vi "Module Loop.vi"(8 "error in (no error)":errorcluster, 11 "GenericGuiAI in":refnum<class "GenericGuiAI.lvclass">) -> (0 "error out":errorcluster, 3 "GenericGuiAI out":refnum<class "GenericGuiAI.lvclass">)   [LabVIEW 2020, in "VolatusDAQGenericGUI.lvlib" / "GenericGuiAI.lvclass"]
uses:
  GenericGuiAI.lvclass
  C:/dev/lv20CE/relink/lv-volatus/Volatus/Module/Module.lvclass
  Volatus/Module/Module.lvclass/Module.ctl
  Volatus/MessageQ/MessageQ.lvclass/MessageQ.ctl
  Volatus/Module/Module.lvclass
  <vilib>/Utility/error.llb/Error Cluster From Error Code.vi
  Volatus/MessageQ/MessageQ.lvclass
panel:
  in  "Tree":string(tree)
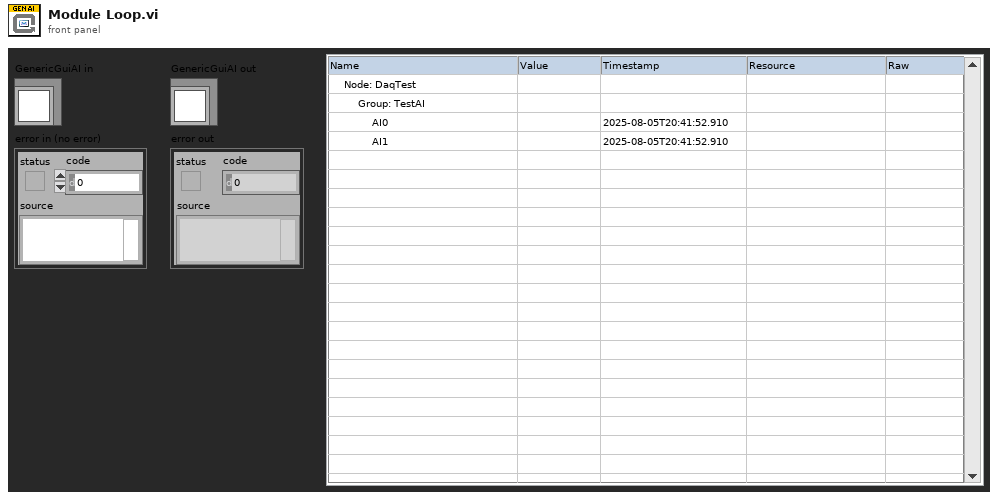
[diagram p1: front panel]
types:
  T1 = enum32{"Invalid", "Standard", "Closed", "Hidden", "Minimized", "Maximized"}
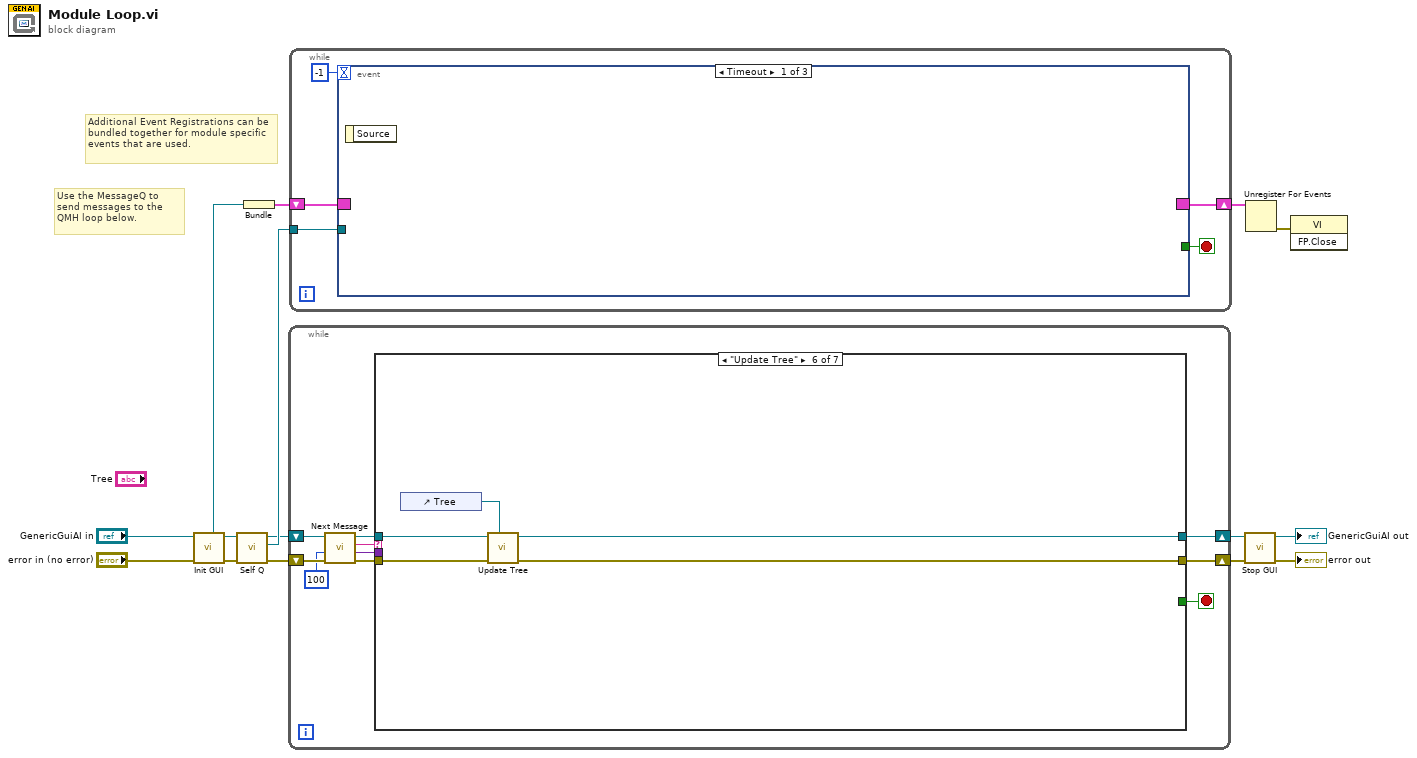
[diagram p0: block diagram]
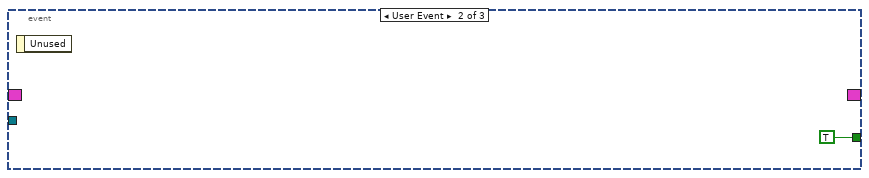
[diagram p2: hidden frame]
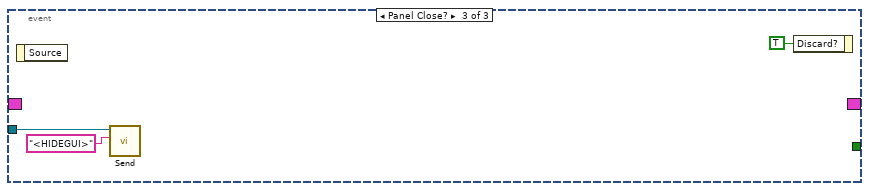
[diagram p3: hidden frame]
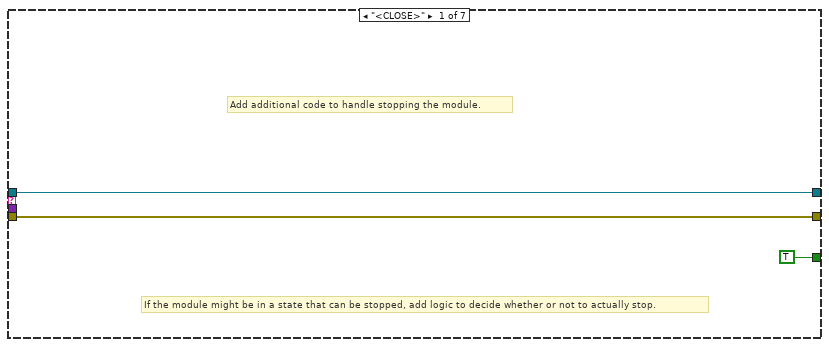
[diagram p4: hidden frame]
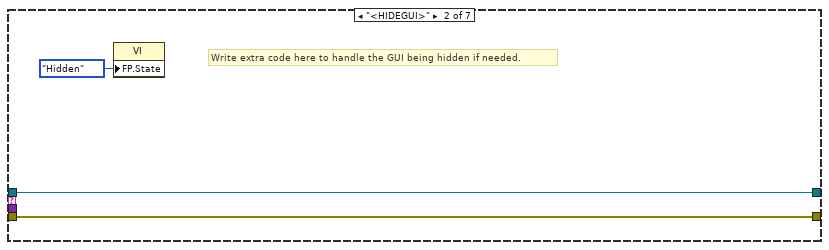
[diagram p5: hidden frame]
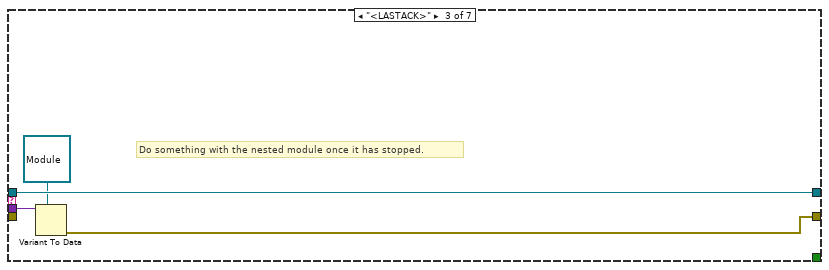
[diagram p6: hidden frame]
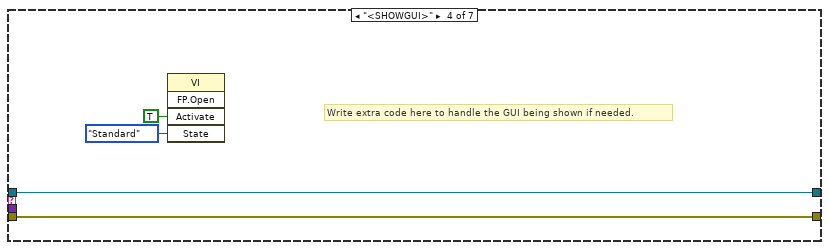
[diagram p7: hidden frame]
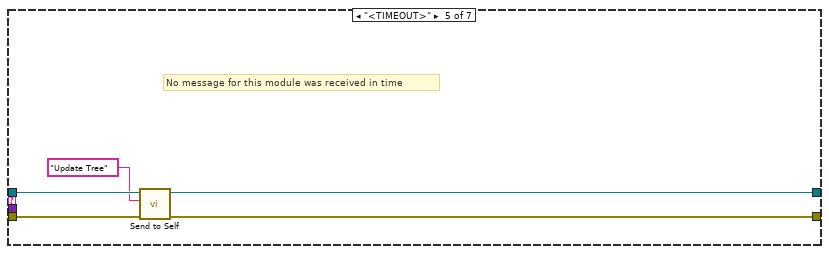
[diagram p8: hidden frame]
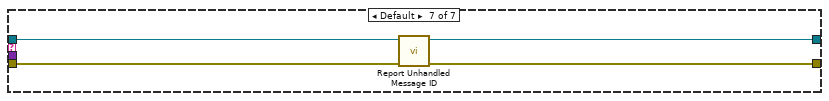
[diagram p9: hidden frame]
diagram:
  # "Additional Event Registrations can be bundled together for module specific events that are used."
  # "Use the MessageQ to send messages to the QMH loop below."
  n1 = call "Init GUI.vi"("Module in"="GenericGuiAI in") -> ("Module out"=w7:refnum<class "GenericGuiAI.lvclass">, "Event Reg"=w12:refnum<event-registration>)  [unwired: 9 in]
  n2 = call "Self Q.vi"("Module in"=w7) -> ("Self Q"=w6:refnum<class "MessageQ.lvclass">, "Module out"=w5:refnum<class "GenericGuiAI.lvclass">)  [unwired: 9 in]
  n3 = Bundle("Event Reg"=w12) -> (w8:cluster{"Event Reg":refnum<event-registration>})  [unwired: 1 in]
  n4 = while {
    shift-right: [w18] -> w10
    shift-left: w5 -> [w23]
    shift-right: [w17] -> w11
    shift-left: "error in (no error)" -> [w22]
    stop <- w16 stop-if-true
    n5 = call "Next Message.vi"("error in (no error)"=w22, "Timeout ms (-1)"=100, "Module in"=w23) -> ("error out"=w21:errorcluster, "Data"=w15:variant, "ID"=w20:string, "Module out"=w19:refnum<class "GenericGuiAI.lvclass">)  [unwired: 5 in]
    n6 = case shown="\"Update Tree\"" w20 {
      tunnel: w21 -> [w24 w28 _ w36 w42 w47 w51]
      tunnel: w19 -> [w25 w29 w33 w37 w40 w45 w49]
      tunnel: [w25 w29 w33 w37 w39 w44 w48] -> w18
      tunnel: [w24 w28 w30 w36 w41 w46 w50] -> w17
      tunnel: [TRUE _ _ _ _ _ _] -> w16
      tunnel: w15 -> [_ _ w32 _ _ _ _]
      frame "<CLOSE>" {
        # "If the module might be in a state that can be stopped, add logic to decide whether or not to actually stop."
        # "Add additional code to handle stopping the module."
      }
      frame "<HIDEGUI>" {
        # "Write extra code here to handle the GUI being hidden if needed."
        n7 = property class="VI"("FP.State"=T1."Hidden" ("Front Panel Window:State")) -> ()  [unwired: 2 in, 2 out]
      }
      frame "<LASTACK>" {
        # "Do something with the nested module once it has stopped."
        n8 = Variant To Data(type=refnum<class "Module.lvclass"> refnum ("Volatus:Module"), Variant=w32) -> (error out=w30:errorcluster)  [unwired: 1 in, 1 out]
      }
      frame "<SHOWGUI>" {
        # "Write extra code here to handle the GUI being shown if needed."
        n9 = invoke class="VI" method="FP.Open"("Activate"=TRUE ("Activate?"), "State"=T1."Standard") -> ()  [unwired: 3 in, 5 out]
      }
      frame "<TIMEOUT>" {
        # "No message for this module was received in time"
        n10 = call "Send to Self.vi"("error in (no error)"=w42, "Message ID"="Update Tree", "Module in"=w40) -> ("error out"=w41:errorcluster, "Module out"=w39:refnum<class "GenericGuiAI.lvclass">)  [unwired: 7 in]
      }
      frame "Update Tree" {
        n11 = control-ref of="Tree"() -> (w43:refnum<vi>)
        n12 = call "Update Tree.vi"("Tree"=w43, "error in (no error)"=w47, "GenericGuiAI in"=w45) -> ("error out"=w46:errorcluster, "GenericGuiAI out"=w44:refnum<class "GenericGuiAI.lvclass">)  [unwired: 7 in]
      }
      frame Default {
        n13 = call "Report Unhandled Message ID.vi"("error in (no error)"=w51, "Module in"=w49) -> ("error out"=w50:errorcluster, "Module out"=w48:refnum<class "GenericGuiAI.lvclass">)  [unwired: 8 in]
      }
    }
  }
  n14 = while {
    tunnel: w6 -> [w56]
    shift-right: [w54] -> w9
    shift-left: w8 -> [w55]
    stop <- w53 stop-if-true
    n15 = event shown="[0] Timeout" {
      selector: w55 -> [_ _ _]
      dyn-events: [_ _ _] -> w54
      timeout: -1 -> [_ _ _]
      tunnel: w56 -> [_ _ w59]
      tunnel: [_ TRUE _] -> w53
      event Timeout {
        n16 = event-data() -> ()  [unwired: 1 in, 1 out]
      }
      event User Event {
        n17 = event-data() -> ()  [unwired: 1 in, 1 out]
      }
      event Panel Close? {
        n18 = event-data() -> ()  [unwired: 1 in, 1 out]
        n19 = call "Send.vi"("ID"="<HIDEGUI>", "MessageQ in"=w59) -> ()  [unwired: 8 in, 2 out]
        n20 = event-data("Discard?"=TRUE) -> ()  [unwired: 1 in, 1 out]
      }
    }
  }
  n21 = call "Stop GUI.vi"("error in (no error)"=w11, "Module in"=w10) -> ("error out"=→"error out":errorcluster, "Module out"=→"GenericGuiAI out":refnum<class "GenericGuiAI.lvclass">)  [unwired: 8 in]
  n22 = Unregister For Events(event registration refnum=w9) -> (error out=w13:errorcluster)  [unwired: 1 in]
  n23 = invoke class="VI" method="FP.Close"(error in=w13) -> ()  [unwired: 2 in, 3 out]
